vi "Init.vi"(8 "error in (no error)":errorcluster, 11 "Delta Param":T1={"f"=0.4763, "e"=0.1628, "rf"=0.2, "re"=0.626}) -> (0 "error out":errorcluster, 3 "Delta Robot Kin":refnum<class "Delta Robot Kinematics.lvclass">)   [LabVIEW 2013, in "Delta Robot Kinematics.lvclass"]
uses:
  Delta Robot Kinematics.lvclass
  Delta Robot Param.ctl
  Delta Robot Kinematics.lvclass/Delta Robot Kinematics.ctl
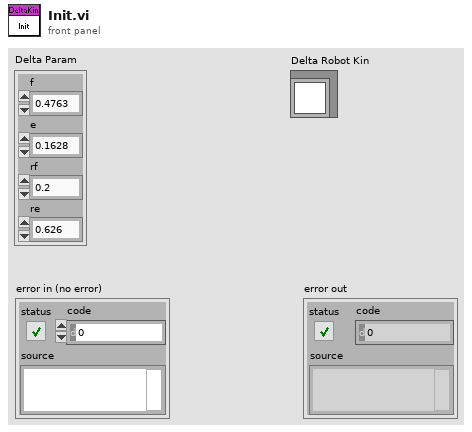
[diagram p1: front panel]
types:
  T1 = typedef "Delta Robot Kinematics.lvclass/Delta Robot Param.ctl" = cluster{"f":dbl, "e":dbl, "rf":dbl, "re":dbl}
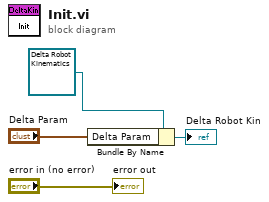
[diagram p0: block diagram]
diagram:
  n1 = Bundle By Name(cluster=refnum<class "Delta Robot Kinematics.lvclass"> refnum ("Delta Robot Kinematics.lvclass"), "Delta Param"="Delta Param") -> (→"Delta Robot Kin":refnum<class "Delta Robot Kinematics.lvclass">)
  "error out" <- "error in (no error)"
